vi "Engine Out - Faults - CAC Outlet Temp.vi"(11 "CAC Outlet Temperature [C]":sgl) -> ()   [LabVIEW 2015, in "ECS-RT.lvlib"]
uses:
  ECS-RT.lvlib
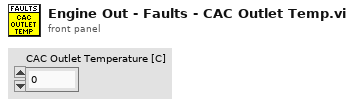
[diagram p1: front panel]
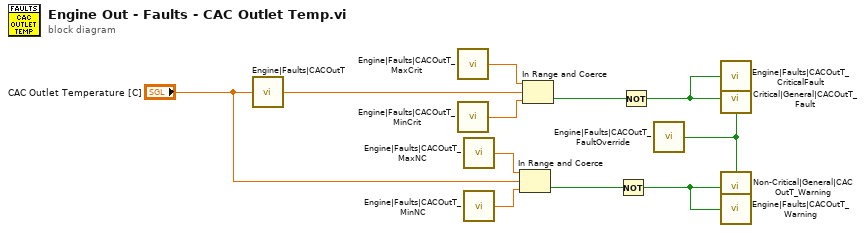
[diagram p0: block diagram]
diagram:
  n1 = call "Engine|Faults|CACOutT"("Value"="CAC Outlet Temperature [C]") -> ()
  n2 = call "Engine|Faults|CACOutT_MaxCrit"() -> ("Value"=w5:sgl)
  n3 = call "Engine|Faults|CACOutT_MinCrit"() -> ("Value"=w4:sgl)
  n4 = call "Engine|Faults|CACOutT_MaxNC"() -> ("Value"=w9:sgl)
  n5 = call "Engine|Faults|CACOutT_MinNC"() -> ("Value"=w8:sgl)
  n6 = In Range and Coerce(upper limit=w9, x="CAC Outlet Temperature [C]", lower limit=w8) -> (In Range?=w7:bool)  [unwired: 1 out]
  n7 = In Range and Coerce(upper limit=w5, x="CAC Outlet Temperature [C]", lower limit=w4) -> (In Range?=w3:bool)  [unwired: 1 out]
  n8 = Not(x=w7) -> (.not. x?=w10:bool)
  n9 = Not(x=w3) -> (.not. x?=w6:bool)
  n10 = call "Engine|Faults|CACOutT_FaultOverride"() -> ("Value"=w1:bool)
  n11 = call "Engine|Faults|CACOutT_CriticalFault"("Value"=w6) -> ()
  n12 = call "Critical|General|CACOutT_Fault"("Fault"=w6, "Override (F)"=w1) -> ()  [unwired: 1 in]
  n13 = call "Non-Critical|General|CACOutT_Warning"("Fault"=w10, "Override (F)"=w1) -> ()  [unwired: 1 in]
  n14 = call "Engine|Faults|CACOutT_Warning"("Value"=w10) -> ()
